vi "GetCurentDateTime.vi"() -> (0 "time":string, 1 "date":string)   [LabVIEW 2010]
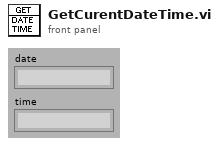
[diagram p1: front panel]
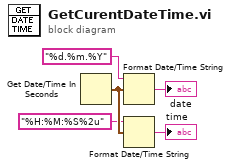
[diagram p0: block diagram]
diagram:
  n1 = Get Date/Time In Seconds() -> (seconds since 1Jan1904=w5:timestamp)
  n2 = Format Date/Time String(time format string (%c)="%d.%m.%Y", seconds (now)=w5) -> (date/time string=→"date":string)  [unwired: 1 in]
  n3 = Format Date/Time String(time format string (%c)="%H:%M:%S%2u", seconds (now)=w5) -> (date/time string=→"time":string)  [unwired: 1 in]
